vi "SteerComand.vi"(8 "Speed":dbl, 11 "SteeringAngle":dbl) -> (2 "ManualActCommand":dbl[](array[numeric]))   [LabVIEW 2012]
doc: "This sub VI takes in a Midbrian steering command (-45>steer<45 degrees)\nand a robot speed (Ft/sec) and loads both into\na 90 slot steering array in preperation for it\nto act as an input to a voting style command arbiter."
uses:
  <vilib>/Analysis/1siggen.llb/Ramp Pattern by Samples.vi
  <vilib>/gmath/statdist.llb/Normal PDF.vi
  <vilib>/Analysis/NI_AALBase.lvlib
  <vilib>/gmath/NI_Gmath.lvlib
panel:
  out "Waveform Graph":dbl[](graph)
  # "This subVI converts a steering wheel\ncommand angle and  robot speed\ninto a voting style array for the\nACT arbiter."
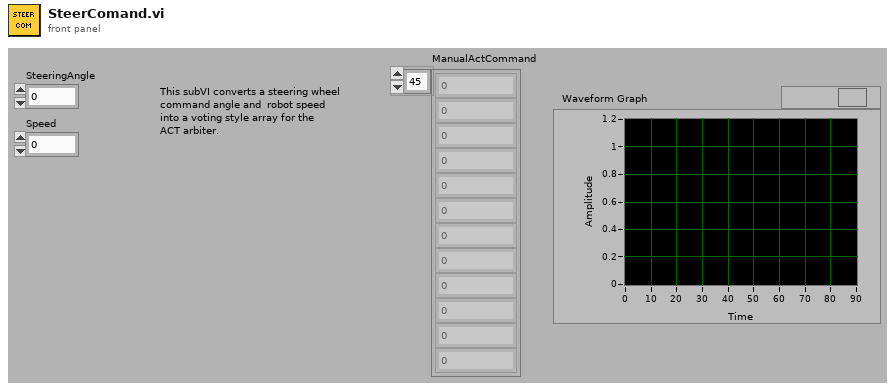
[diagram p1: front panel]
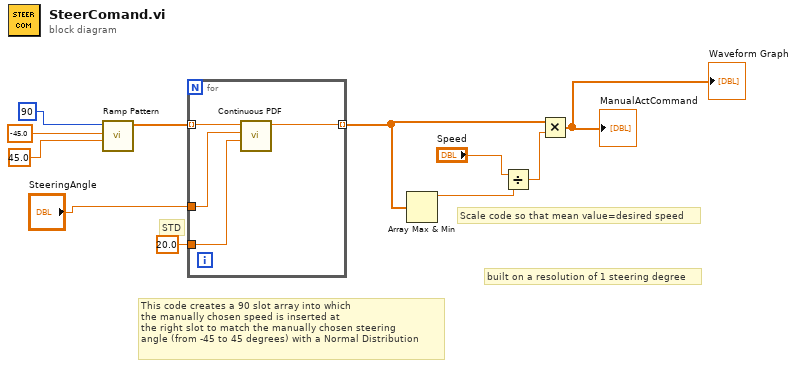
[diagram p0: block diagram]
diagram:
  # "built on a resolution of 1 steering degree"
  # "Scale code so that mean value=desired speed"
  # "STD"
  # "This code creates a 90 slot array into which\nthe manually chosen speed is inserted at\nthe right slot to match the manually chosen steering\nangle (from -45 to 45 degrees) with a Normal Distribution"
  n1 = call-poly <vilib>:"Ramp Pattern.vi"("start"=45.0, "end"=-45.0 ("end (Normal)"), "samples"=90) -> ("Ramp Pattern"=w9:dbl[])  [unwired: 7 in, 1 out]
  n2 = for {
    tunnel: w9 -> [w15] mode=indexing
    tunnel: 20.0 ("std (Normal)") -> [w14]
    tunnel: [w13] -> w3 mode=indexing
    tunnel: "SteeringAngle" -> [w12]
    n3 = call-poly <vilib>:"Continuous PDF.vi"("std"=w14, "mean"=w12, "x"=w15) -> ("pdf(x)"=w13:dbl)  [unwired: 7 in, 1 out]
  }
  n4 = Array Max & Min(array=w3) -> (max value=w6:dbl)  [unwired: 3 out]
  n5 = Divide(x="Speed", y=w6) -> (x/y=w4:dbl)
  n6 = Multiply(x=w3, y=w4) -> (x*y=→"ManualActCommand" →"Waveform Graph":dbl[])
